vi "Format XY Graph.vi"(0 "XYGraph in":refnum<vi>, 1 "Point Style":u8[](array[numeric])=[2, 0, 0], 5 "Plot Interpolation":u8[](array[numeric])=[0, 2, 2], 7 "Plot Color":u32[](array[colorbox])=[2774271, 4587306, 16716354, 65351, 5898088, 3731200], 9 "Plot Name":string[](array[string])=["Measured", "Upper Lim", "Lower Lim"], 11 "error in (no error)":errorcluster, 12 "XY Text":T1={"X Scale.Name Label.Text"="Voltage (V)", "Y Scale.Name Label.Text"="Current (mA)", "Label.Text"="LED Current Consumption"}) -> (4 "XYGraph out":refnum<vi>, 15 "error out":errorcluster)   [LabVIEW 2018]
panel:
  # "Data Input"
  # "Data Output"
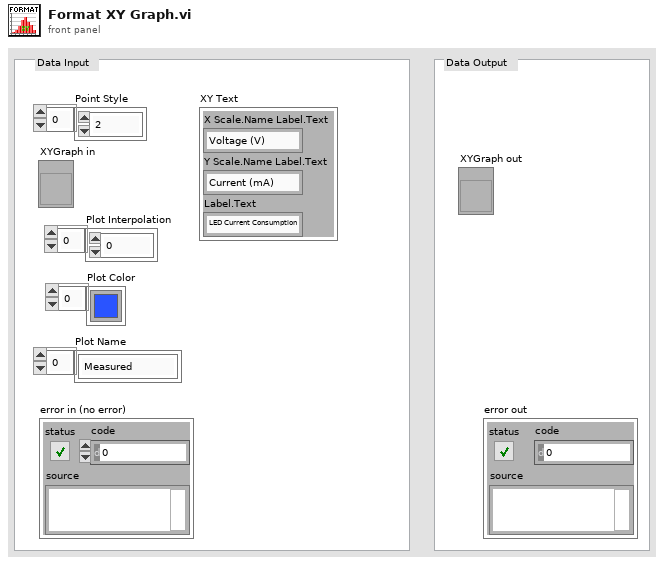
[diagram p1: front panel]
types:
  T1 = cluster{"X Scale.Name Label.Text":string, "Y Scale.Name Label.Text":string, "Label.Text":string}
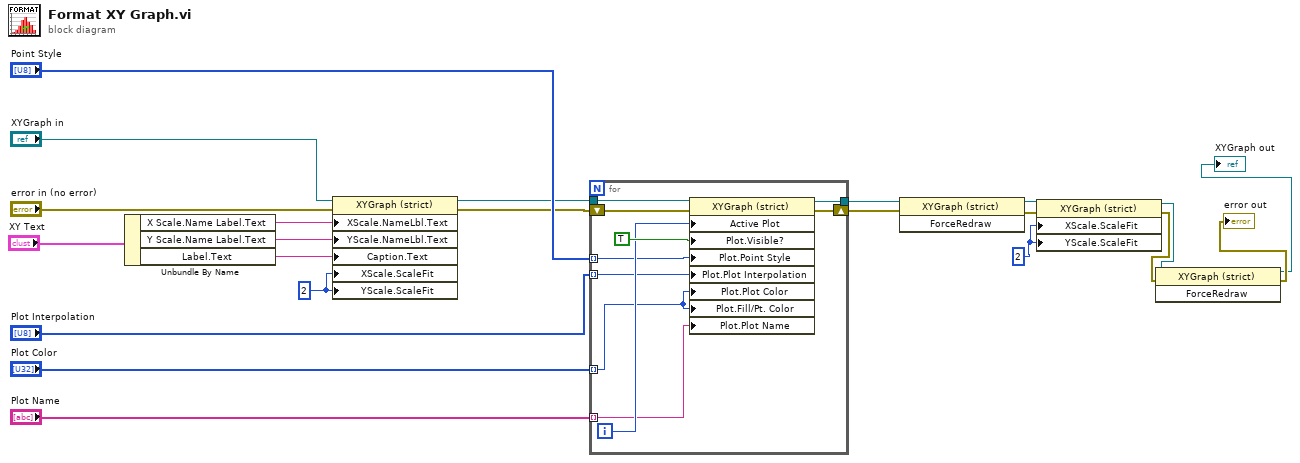
[diagram p0: block diagram]
diagram:
  w5 = u8 2 ("X Scale.Scale Fit")
  w8 = u8 2 ("X Scale.Scale Fit")
  n1 = Unbundle By Name("XY Text") -> ("X Scale.Name Label.Text"=w11:string, "Y Scale.Name Label.Text"=w10:string, "Label.Text"=w9:string)
  n2 = property class="XYGraph (strict)"(reference="XYGraph in", error in="error in (no error)", "XScale.NameLbl.Text"=w11, "YScale.NameLbl.Text"=w10, "Caption.Text"=w9, "XScale.ScaleFit"=w8, "YScale.ScaleFit"=w8) -> (reference out=w14:refnum<vi>, error out=w13:errorcluster)
  n3 = for {
    tunnel: w14 -> [w31]
    tunnel: "Plot Color" -> [w26] mode=indexing
    tunnel: "Plot Interpolation" -> [w27] mode=indexing
    tunnel: "Point Style" -> [w28] mode=indexing
    tunnel: [w29] -> w18
    tunnel: "Plot Name" -> [w25] mode=indexing
    shift-right: [w24] -> w20
    shift-left: w13 -> [w23]
    i -> [w30]
    n4 = property class="XYGraph (strict)"(reference=w31, error in=w23, "Active Plot"=w30, "Plot.Visible?"=TRUE ("Plot.Visible"), "Plot.Point Style"=w28, "Plot.Plot Interpolation"=w27, "Plot.Plot Color"=w26, "Plot.Fill/Pt. Color"=w26, "Plot.Plot Name"=w25) -> (reference out=w29:refnum<vi>, error out=w24:errorcluster)
  }
  n5 = invoke class="XYGraph (strict)" method="ForceRedraw"(reference=w18, error in=w20) -> (reference out=w7:refnum<vi>, error out=w6:errorcluster)  [unwired: 1 in, 1 out]
  n6 = property class="XYGraph (strict)"(reference=w7, error in=w6, "XScale.ScaleFit"=w5, "YScale.ScaleFit"=w5) -> (reference out=w3:refnum<vi>, error out=w4:errorcluster)
  n7 = invoke class="XYGraph (strict)" method="ForceRedraw"(reference=w3, error in=w4) -> (reference out=→"XYGraph out":refnum<vi>, error out=→"error out":errorcluster)  [unwired: 1 in, 1 out]
